vi "AsymmetricDebounce.vi"(1 "Reset":bool, 2 "Input":bool, 3 "DeactivateSamples":i32=10, 4 "ActivateSamples":i32=10) -> (0 "Output":bool)   [LabVIEW 2019, in "ArgosLib.lvlib"]
uses:
  ArgosLib.lvlib
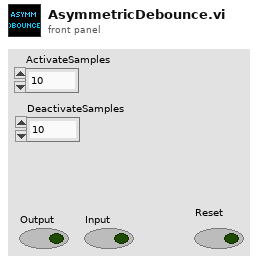
[diagram p1: front panel]
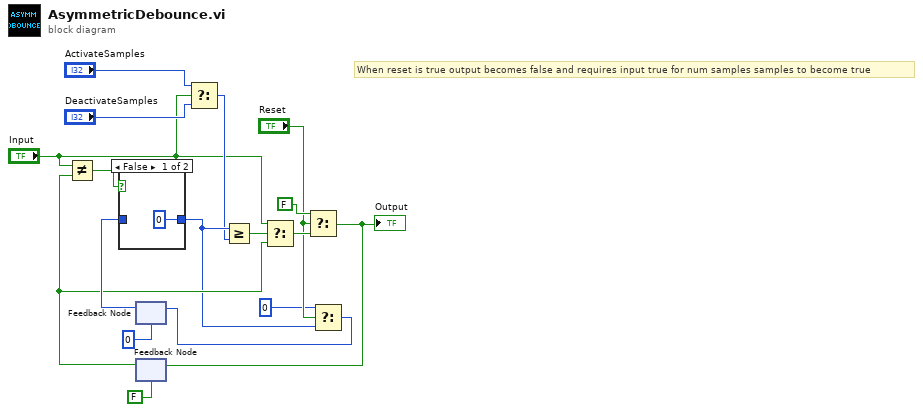
[diagram p0: block diagram]
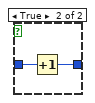
[diagram p2: hidden frame]
diagram:
  # "When reset is true output becomes false and requires input true for num samples samples to become true"
  n1 = feedback #1(0) -> (w15:i32)
  n2 = feedback #2(FALSE ("Input")) -> (w13:bool)
  n3 = Not Equal?(x="Input", y=w13) -> (x != y?=w17:bool)
  n4 = case shown="False" w17 {
    tunnel: w15 -> [_ w20]
    tunnel: [0 w19] -> w8
    frame False {
    }
    frame True {
      n5 = Increment(x=w20) -> (x+1=w19:i32)
    }
  }
  n6 = Select(t="ActivateSamples", s="Input", f="DeactivateSamples") -> (s? t:f=w2:i32)
  n7 = Greater Or Equal?(x=w8, y=w2) -> (x >= y?=w16:bool)
  n8 = Select(t="Input", s=w16, f=w13) -> (s? t:f=w10:bool)
  n9 = Select(t=FALSE, s="Reset", f=w10) -> (s? t:f=w11:bool)
  "Output" <- w11
  n10 = feedback-in #2(w11) -> ()
  n11 = Select(t=0, s="Reset", f=w8) -> (s? t:f=w5:i32)
  n12 = feedback-in #1(w5) -> ()
